vi "Threshold Results.vi"(4 "Th-L-OC":dbl format="%#_3g", 6 "Th-Low":dbl, 7 "file path (dialog if empty)":path, 8 "Th-H-OC":dbl format="%#_3g", 9 "ET-Delay-SD":dbl, 10 "Th-High":dbl, 11 "Estimated Propagation Delay":dbl) -> ()   [LabVIEW 2014]
doc: "This VI displays the results of threshold value and propagation delay analysis. \n\nDesigned by HB\nhaba@dtu.dk"
uses:
  <vilib>/Utility/file.llb/Write To Spreadsheet File (string).vi
panel:
  out "Estimated Propagation Delay":string
  in  "OK":bool
  # "±"
  # "Results of Threshold Value Analysis"
  # "Estimated Threshold Values"
  # "Output Consistency (%)"
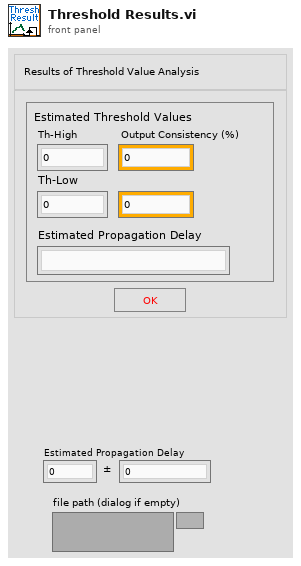
[diagram p1: front panel]
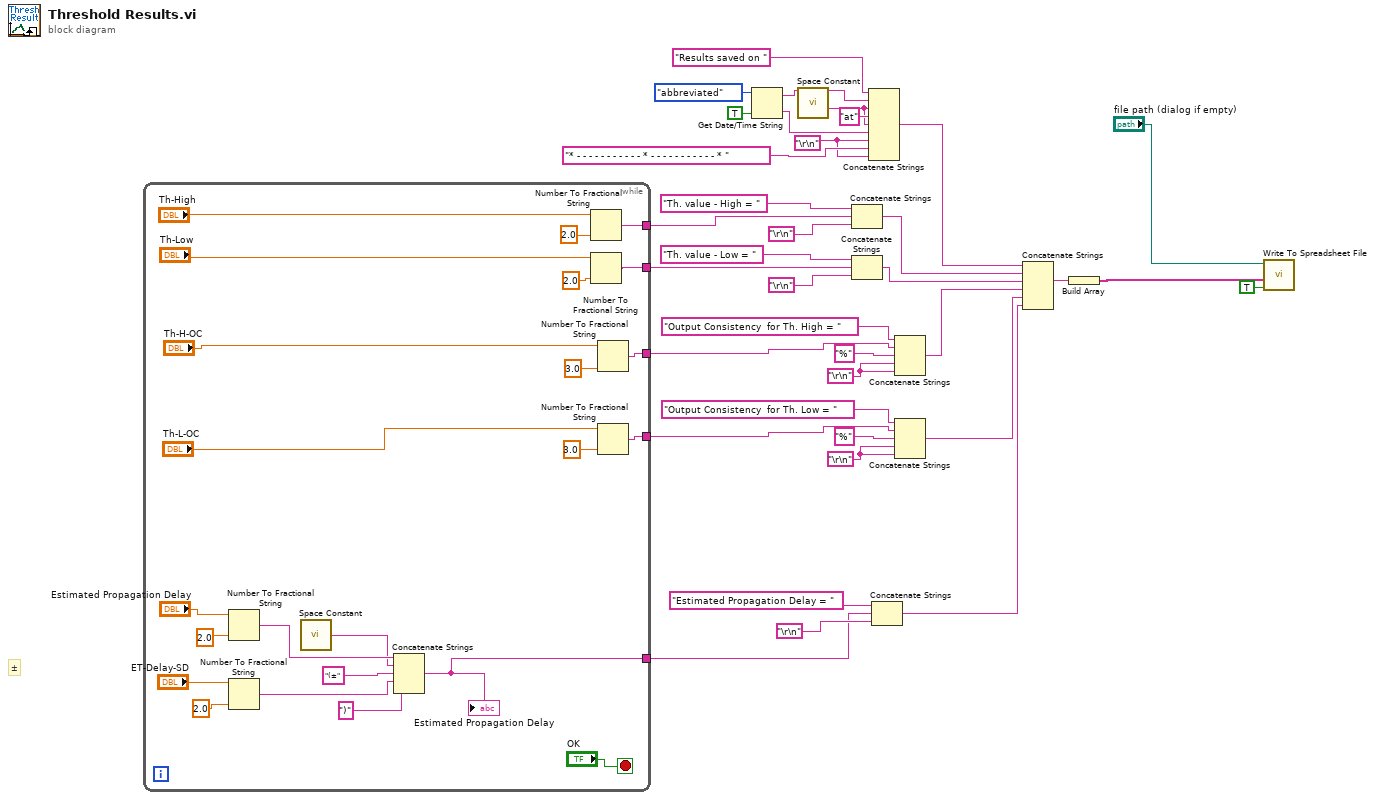
[diagram p0: block diagram]
diagram:
  w5 = "\r\n"
  w13 = "\r\n"
  w15 = "\r\n"
  # "±"
  n1 = while {
    tunnel: [w50] -> w33
    tunnel: [w49] -> w30
    tunnel: [w47] -> w27
    tunnel: [w45] -> w9
    tunnel: [w44] -> w4
    stop <- "OK" stop-if-true
    n2 = Number To Fractional String(number="Estimated Propagation Delay", precision (6)=2.0) -> (F-format string=w57:string)  [unwired: 2 in]
    n3 = Number To Fractional String(number="ET-Delay-SD", precision (6)=2.0) -> (F-format string=w53:string)  [unwired: 2 in]
    n4 = call <vilib>:"Space Constant.vi"() -> ("String"=w55:string)
    n5 = Concatenate Strings(w57, w55, "(±" ("String"), w53, ")" ("String")) -> (w49:string)
    "Estimated Propagation Delay" <- w49
    n6 = Number To Fractional String(number="Th-High", precision (6)=2.0) -> (F-format string=w50:string)  [unwired: 2 in]
    n7 = Number To Fractional String(number="Th-Low", precision (6)=2.0) -> (F-format string=w45:string)  [unwired: 2 in]
    n8 = Number To Fractional String(number="Th-H-OC", precision (6)=3.0) -> (F-format string=w47:string)  [unwired: 2 in]
    n9 = Number To Fractional String(number="Th-L-OC", precision (6)=3.0) -> (F-format string=w44:string)  [unwired: 2 in]
  }
  n10 = Get Date/Time String(date format (0)=enum16{"short", "long", "abbreviated"}."abbreviated", want seconds? (F)=TRUE) -> (date string=w22:string, time string=w19:string)  [unwired: 1 in]
  n11 = call <vilib>:"Space Constant.vi"() -> ("String"=w20:string)
  n12 = Concatenate Strings("Th. value - High = ", w33, "\r\n") -> (w26:string)
  n13 = Concatenate Strings("Th. value - Low = ", w9, "\r\n") -> (w8:string)
  n14 = Concatenate Strings("Results saved on " ("string"), w22, w20, "at" ("string"), w20, w19, w13, "* - - - - - - - - - - - * - - - - - - - - - - - * " ("string"), w13) -> (w16:string)
  n15 = Concatenate Strings("Estimated Propagation Delay = ", w30, "\r\n") -> (w6:string)
  n16 = Concatenate Strings("Output Consistency  for Th. High = ", w27, "%" ("string"), w15, w15) -> (w7:string)
  n17 = Concatenate Strings("Output Consistency  for Th. Low = ", w4, "%" ("string"), w5, w5) -> (w1:string)
  n18 = Concatenate Strings(w16, w26, w8, w7, w1, w6) -> (w25:string)
  n19 = Build Array(w25) -> (w24:string[])
  n20 = call-poly <vilib>:"Write To Spreadsheet File.vi"("append to file? (new file:F)"=TRUE, "1D data"=w24, "file path (dialog if empty)"="file path (dialog if empty)") -> ()  [unwired: 5 in, 1 out]
